vi "Put Block List.vi"(5 "Uncommitted Blocks":string[](array[string]), 6 "Latest Blocks":string[](array[string]), 7 "Committed Blocks":string[](array[string]), 8 "error in (no error)":errorcluster, 9 "Blob":string, 10 "Container":string, 11 "Azure Session in":refnum<class "Session.lvclass">) -> (0 "error out":errorcluster, 3 "Azure Session out":refnum<class "Session.lvclass">)   [LabVIEW 2015, in "NI_Azure_Blob.lvlib"]
doc: "Commits a blob by specifying the set of block IDs that comprise the block blob."
uses:
  NI_Azure_Blob.lvlib
  Core/Session/Session.lvclass
  Core/Name Value Pair.ctl
  Core/Session/Session.lvclass/Session.ctl
  Core/Session/Write Request Parameters.vi
  Core/Session/Write HTTP Verb.vi
  Core/Session/Write URL Suffix.vi
  Core/Session/Write Request body.vi
  Core/NI_Azure_Core.lvlib
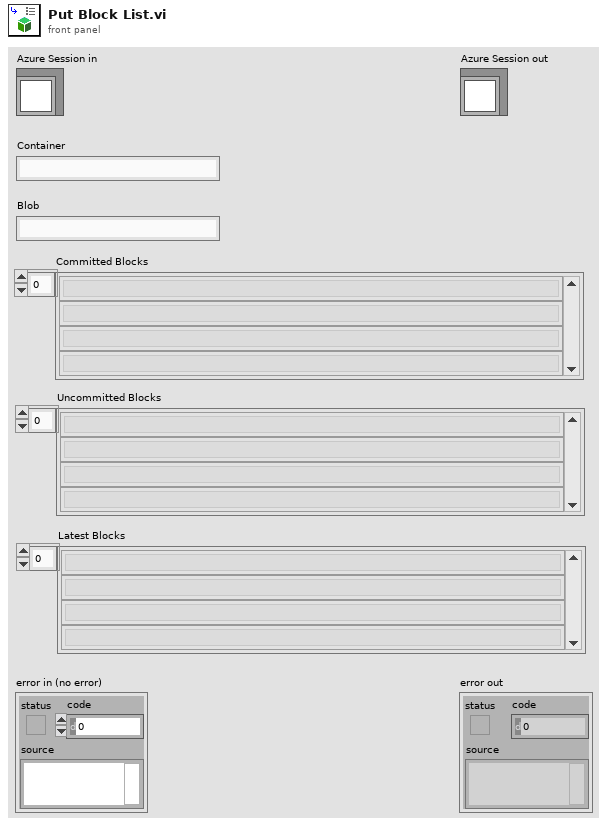
[diagram p1: front panel]
types:
  T1 = typedef "NI_Azure_Core.lvlib/Name Value Pair.ctl" = cluster{"name":string, "value":string}
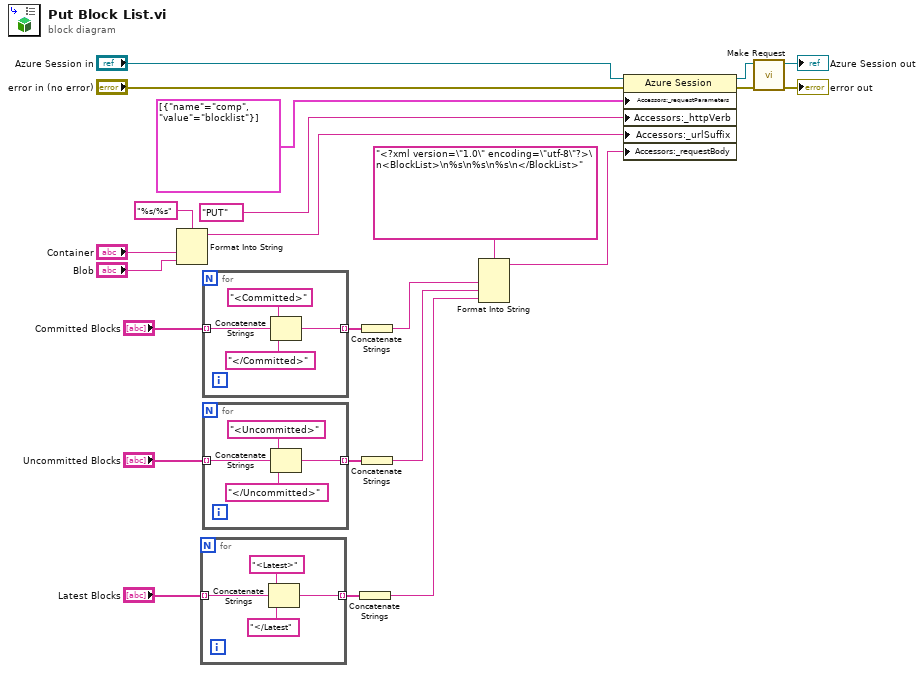
[diagram p0: block diagram]
diagram:
  n1 = Format Into String(format string="%s/%s", "Container", "Blob") -> (resulting string=w13:string)  [unwired: 2 in, 1 out]
  n2 = for {
    tunnel: "Latest Blocks" -> [w27] mode=indexing
    tunnel: [w24] -> w5 mode=indexing
    n3 = Concatenate Strings("<Latest>", w27, "</Latest") -> (w24:string)
  }
  n4 = for {
    tunnel: "Committed Blocks" -> [w31] mode=indexing
    tunnel: [w28] -> w8 mode=indexing
    n5 = Concatenate Strings("<Committed>", w31, "</Committed>") -> (w28:string)
  }
  n6 = for {
    tunnel: "Uncommitted Blocks" -> [w35] mode=indexing
    tunnel: [w32] -> w6 mode=indexing
    n7 = Concatenate Strings("<Uncommitted>", w35, "</Uncommitted>") -> (w32:string)
  }
  n8 = Concatenate Strings(w5) -> (w1:string)
  n9 = Concatenate Strings(w8) -> (w7:string)
  n10 = Concatenate Strings(w6) -> (w4:string)
  n11 = Format Into String(format string="<?xml version=\"1.0\" encoding=\"utf-8\"?>\n<BlockList>\n%s\n%s\n%s\n</BlockList>", w7, w4, w1) -> (resulting string=w10:string)  [unwired: 2 in, 1 out]
  n12 = property class="Azure Session"(reference="Azure Session in", error in="error in (no error)", "Accessors:_requestParameters"=T1[] [{"name"="comp", "value"="blocklist"}] ("appended array"), "Accessors:_httpVerb"="PUT" ("HTTP-Verb"), "Accessors:_urlSuffix"=w13, "Accessors:_requestBody"=w10) -> (reference out=w17:refnum<class "Session.lvclass">, error out=w15:errorcluster)
  n13 = call "Make Request.vi"("error in (no error)"=w15, "Session in"=w17) -> ("error out"=→"error out":errorcluster, "Session out"=→"Azure Session out":refnum<class "Session.lvclass">)  [unwired: 7 in, 1 out]
